vi "Set Array Size.vi"(4 "Default":string, 5 "Key name":string, 6 "Index":i32=4, 7 "Section name":string, 8 "error in (no error)":errorcluster, 9 "Use Key Regex? [F]":bool, 10 "Use Section Regex? [F]":bool, 11 "Carya Config in":refnum<class "Carya Config.lvclass">) -> (0 "error out":errorcluster, 3 "Carya Config out":refnum<class "Carya Config.lvclass">)   [LabVIEW 2013, in "Carya Config.lvclass"]
doc: "Copyright 2018, Carya Automatisering, Wiebe Walstra."
uses:
  Carya Config.lvclass
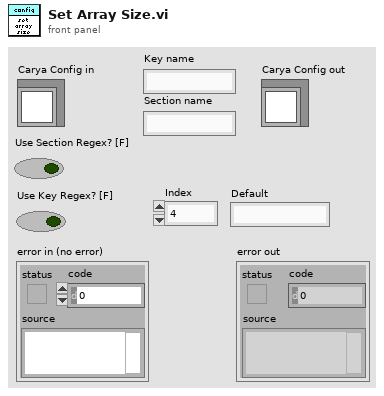
[diagram p1: front panel]
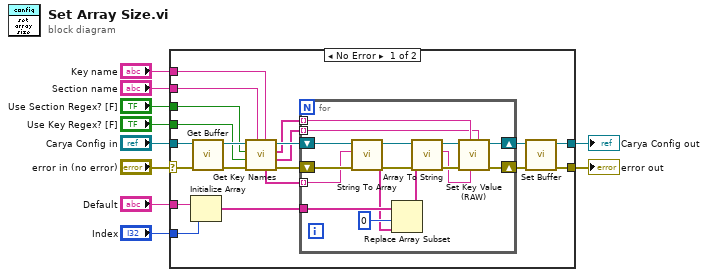
[diagram p0: block diagram]
diagram:
  n1 = case shown="No Error" "error in (no error)" {
    selector: "error in (no error)" -> [w30 w48]
    tunnel: [w20 w48] -> w9
    tunnel: [w18 w47] -> w7
    tunnel: "Carya Config in" -> [w12 w47]
    tunnel: "Section name" -> [w24 _]
    tunnel: "Key name" -> [w23 _]
    tunnel: "Use Section Regex? [F]" -> [w22 _]
    tunnel: "Use Key Regex? [F]" -> [w21 _]
    tunnel: "Index" -> [w27 _]
    tunnel: "Default" -> [w11 _]
    frame No Error {
      n2 = Initialize Array(w11, w27) -> (w15:string[])
      n3 = call-dynamic "Get Buffer.vi"("error in (no error)"=w30, "Carya Config in"=w12) -> ("error out"=w29:errorcluster, "Config"=w28:refnum<class "Carya Config.lvclass">)  [unwired: 8 in]
      n4 = call-dynamic "Get Key Names.vi"("Key name/Regex"=w23, "Section name/Regex"=w24, "error in (no error)"=w29, "Use Key Regex? [F]"=w21, "Use Section Regex? [F]"=w22, "Carya Config in"=w28) -> ("error out"=w17:errorcluster, "Key names"=w13:string[], "Section names"=w14:string[], "Carya Config out"=w25:refnum<class "Carya Config.lvclass">, "Context (concatenated)"=w16:string[])  [unwired: 1 in]
      n5 = for {
        shift-right: [w45] -> w19
        shift-left: w25 -> [w40]
        shift-right: [w46] -> w26
        shift-left: w17 -> [w44]
        tunnel: w16 -> [w39] mode=indexing
        tunnel: w15 -> [w42]
        tunnel: w14 -> [w32] mode=indexing
        tunnel: w13 -> [w31] mode=indexing
        n6 = call-dynamic "String To Array.vi"("error in (no error)"=w44, "resulting string"=w39, "Registry Object"=w40) -> ("error out"=w41:errorcluster, "Array"=w38:string[], "Registry Object"=w36:refnum<class "Carya Config.lvclass">)  [unwired: 6 in]
        n7 = Replace Array Subset(array=w42, new element=w38, index=0) -> (w34:string[])
        n8 = call-dynamic "Array To String.vi"("error in (no error)"=w41, "Array"=w34, "Registry Object"=w36) -> ("error out"=w37:errorcluster, "resulting string"=w33:string, "Registry Object"=w35:refnum<class "Carya Config.lvclass">)  [unwired: 6 in]
        n9 = call-dynamic "Set Key Value (RAW).vi"("Key name"=w31, "Key value"=w33, "Section name"=w32, "error in (no error)"=w37, "Carya Config in"=w35) -> ("error out"=w46:errorcluster, "Carya Config out"=w45:refnum<class "Carya Config.lvclass">)  [unwired: 2 in, 3 out]
      }
      n10 = call-dynamic "Set Buffer.vi"("error in (no error)"=w26, "Carya Config"=w19) -> ("error out"=w20:errorcluster, "Carya Config out"=w18:refnum<class "Carya Config.lvclass">)  [unwired: 8 in]
    }
    frame Error {
    }
  }
  "error out" <- w9
  "Carya Config out" <- w7
